vi "74HC153(或74HC138)和74HC00设计全加器.vi"() -> ()   [LabVIEW 2018]
panel:
  in  "结束":bool
  out "C1":bool
  out "S1":bool
  in  "C0":bool
  in  "B1":bool
  in  "A1":bool
  # "74HC153：双四选一\n74HC00：与非门"
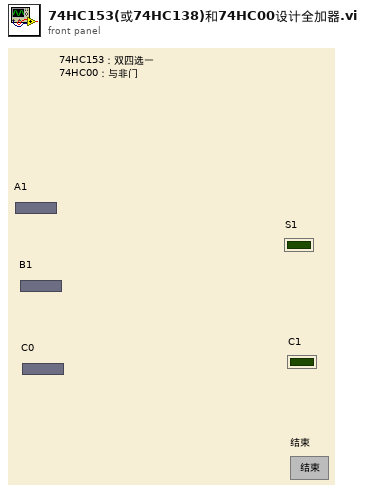
[diagram p1: front panel]
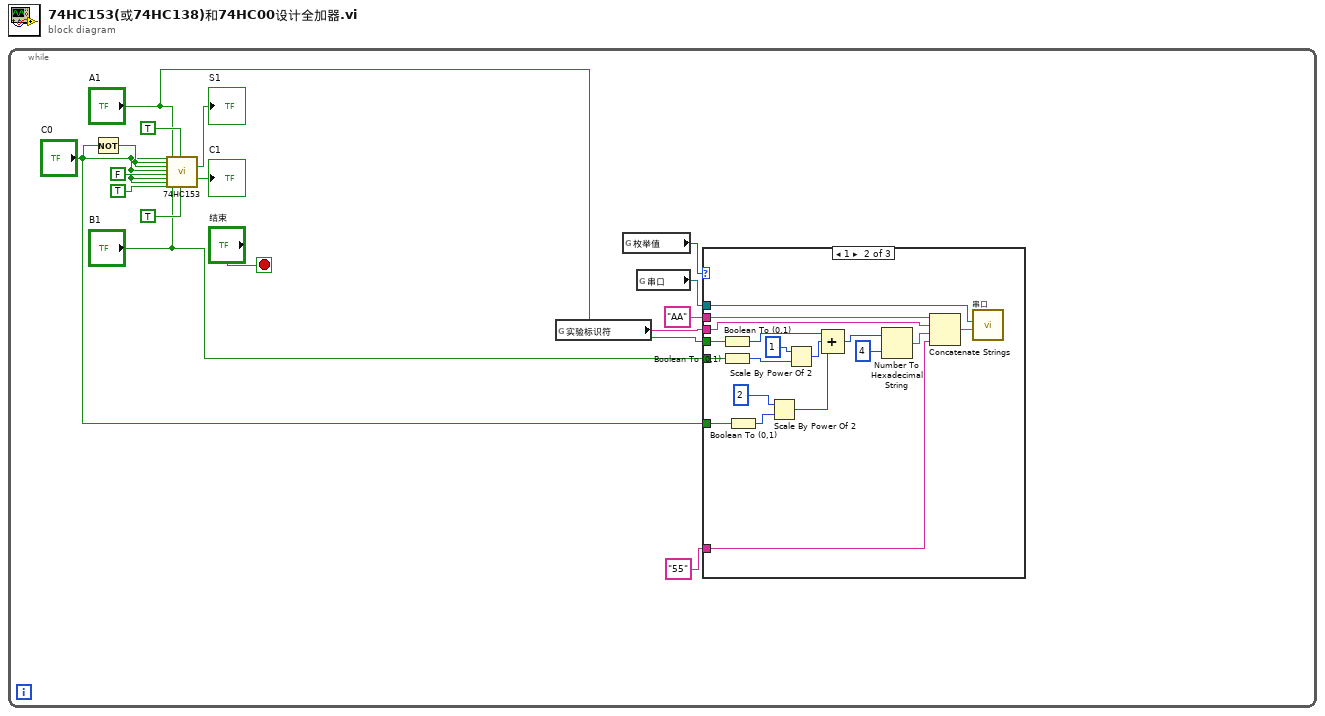
[diagram p0: block diagram]
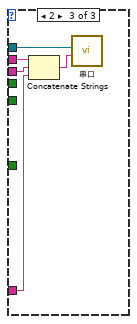
[diagram p3: hidden frame]
diagram:
  n1 = while {
    stop <- "结束" stop-if-true
    n2 = Not(x="C0") -> (.not. x?=w12:bool)
    n3 = call "74HC153.vi"("D10"="C0", "D11"=w12, "D12"=w12, "D13"="C0", "D20"=FALSE, "D21"="C0", "D22"="C0", "D23"=TRUE, "S0"="A1", "S1"="B1", "EN1"=TRUE, "EN2"=TRUE) -> ("Y1"=→"S1":bool, "Y2"=→"C1":bool)  [unwired: 14 in]
    n4 = global read "全局变量.vi" "实验标识符"() -> (w6:string)
    n5 = global read "全局变量.vi" "枚举值"() -> (w8:i8)
    n6 = global read "全局变量.vi" "串口"() -> (w7:refnum<visa-resource-name>)
    n7 = case shown="1" w8 {
      tunnel: "B1" -> [_ w29 _]
      tunnel: "A1" -> [_ w28 _]
      tunnel: w7 -> [_ w27 w37]
      tunnel: w6 -> [_ w26 w38]
      tunnel: "55" -> [_ w25 w35]
      tunnel: "AA" -> [_ w24 w36]
      tunnel: "C0" -> [_ w18 _]
      frame 0, Default {
      }
      frame 1 {
        n8 = Boolean To (0,1)(Boolean=w28) -> (0, 1=w33:i16)
        n9 = Boolean To (0,1)(Boolean=w29) -> (0, 1=w31:i16)
        n10 = Boolean To (0,1)(Boolean=w18) -> (0, 1=w19:i16)
        n11 = Scale By Power Of 2(n=2, x=w19) -> (x*2^n=w20:i16)
        n12 = Scale By Power Of 2(n=1, x=w31) -> (x*2^n=w32:i16)
        n13 = Compound Arithmetic op=ADD ("复合运算")(w33, w32, w20) -> (w23:i16)
        n14 = Number To Hexadecimal String(1:4, 2:w23) -> (0:w21:string)
        n15 = Concatenate Strings(w24, w26, w21, w25) -> (w34:string)
        n16 = call "串口.vi"("字符串"=w34, "VISA resource name"=w27) -> ()  [unwired: 10 in]
      }
      frame 2 {
        n17 = Concatenate Strings(w36, w38, w35) -> (w39:string)
        n18 = call "串口.vi"("字符串"=w39, "VISA resource name"=w37) -> ()  [unwired: 10 in]
      }
    }
  }
